vi "iradon_C (SubVI).vi"(6 "N_rot":dbl=40.0, 7 "N_det":dbl=40.0, 9 "2-D Array of Real":dbl[][](array[numeric])) -> (2 "Intensity Graph 2":dbl[][](graph), 3 "Intensity Graph":dbl[][](graph))   [LabVIEW 2018]
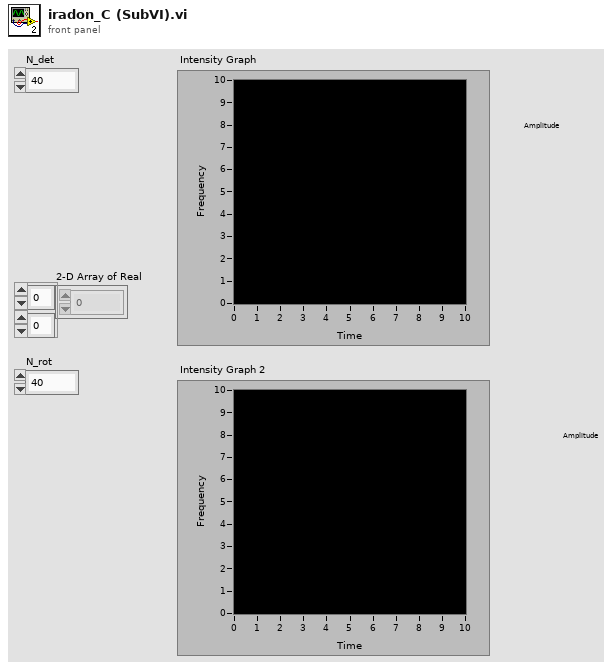
[diagram p1: front panel]
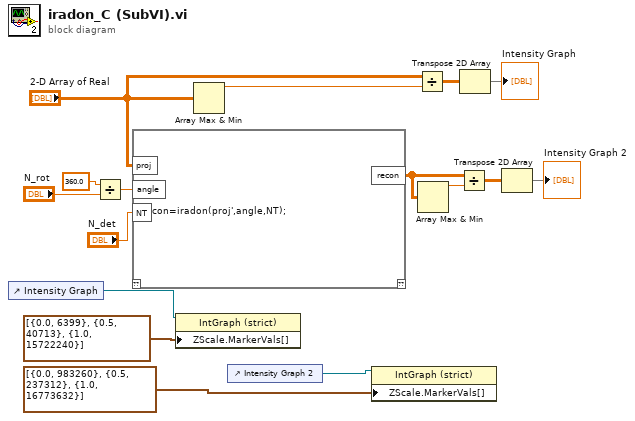
[diagram p0: block diagram]
diagram:
  n1 = control-ref of="Intensity Graph"() -> (w2:refnum<vi>)
  n2 = Divide(x=360.0, y="N_rot") -> (x/y=w3:dbl)
  n3 = script code="recon=iradon(proj',angle,NT);"("proj"="2-D Array of Real", "angle"=w3, "NT"="N_det") -> ("recon"=w15:dbl[][])  [unwired: 1 in, 1 out]
  n4 = property on="Property Node" class="IntGraph (strict)"(reference=w2, "ZScale.MarkerVals[]"=cluster{dbl, u32}[] [{0.0, 6399}, {0.5, 40713}, {1.0, 15722240}] ("Z Scale.Marker Values[]")) -> ()  [unwired: 1 in, 2 out]
  n5 = Array Max & Min(array="2-D Array of Real") -> (max value=w9:dbl)  [unwired: 3 out]
  n6 = control-ref of="Intensity Graph 2"() -> (w1:refnum<vi>)
  n7 = property on="Property Node" class="IntGraph (strict)"(reference=w1, "ZScale.MarkerVals[]"=cluster{dbl, u32}[] [{0.0, 983260}, {0.5, 237312}, {1.0, 16773632}] ("Z Scale.Marker Values[]")) -> ()  [unwired: 1 in, 2 out]
  n8 = Divide(x="2-D Array of Real", y=w9) -> (x/y=w11:dbl[][])
  n9 = Array Max & Min(array=w15) -> (max value=w16:dbl)  [unwired: 3 out]
  n10 = Divide(x=w15, y=w16) -> (x/y=w13:dbl[][])
  n11 = Transpose 2D Array(2D array=w11) -> (transposed array=→"Intensity Graph":dbl[][])
  n12 = Transpose 2D Array(2D array=w13) -> (transposed array=→"Intensity Graph 2":dbl[][])
